vi "Pre-Build Custom Action.vi"() -> (0 "error out":errorcluster)   [LabVIEW 2021]
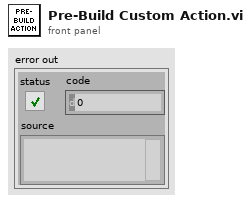
[diagram p1: front panel]
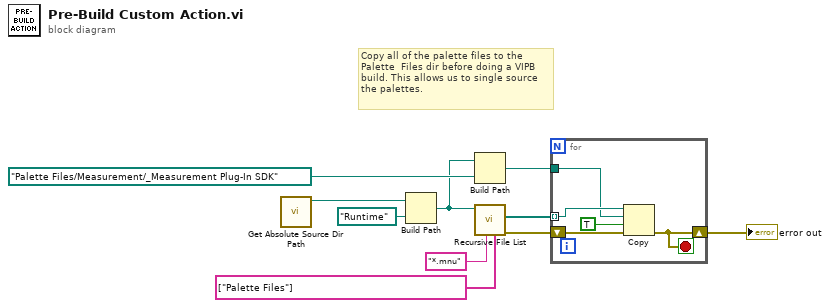
[diagram p0: block diagram]
diagram:
  # "Copy all of the palette files to the \nPalette  Files dir before doing a VIPB\nbuild. This allows us to single source\nthe palettes."
  n1 = call "Get Absolute Source Dir Path.vi"() -> ("source dir"=w1:path)  [unwired: 11 in]
  n2 = Build Path(base path=w1, name or relative path=path "Runtime") -> (appended path=w3:path)
  n3 = Build Path(base path=w3, name or relative path=path "Palette Files/Measurement/_Measurement Plug-In SDK") -> (appended path=w2:path)
  n4 = call <vilib>:"Recursive File List.vi"("Folders to Exclude"=string[] ["Palette Files"], "pattern"="*.mnu", "Folder Path"=w3) -> ("error out"=w6:errorcluster, "All Files in Dir"=w7:path[])  [unwired: 4 in, 3 out]
  n5 = for {
    tunnel: w7 -> [w13] mode=indexing
    tunnel: w2 -> [w12]
    shift-right: [w11] -> w4
    shift-left: w6 -> [w15]
    stop <- w11 stop-if-true
    n6 = Copy(8:w15, 9:TRUE ("overwrite (F)"), 10:w12, 11:w13) -> (0:w11:errorcluster)  [unwired: 1 in, 2 out]
  }
  "error out" <- w4
